vi "log analysis_gps.vi"() -> ()   [LabVIEW 2019] (continued)
0.0344,0.0343,0.0312,0.0792,0.0802,5.0949,0f000005,0*2ff36e63\n\t", "INSPVAXA,USB3,0,49.0,FINESTEERING,2107,283226.350,02000000,471d,15824;INS_ALIGNMENT_COMPLETE,INS_RTKFIXED,37.37108844765,126.72336703725,8.2202,22.3000,0.1175,-0.3192,-0.0049,-0.452699232,-0.802169824,288.131784608,0.2162,0.1626,0.2698,0.0571,0.0479,0.0400,0.0831,0.0841,5.0965,0f000001,0*8912b163\n\t", "INSPVAXA,USB3,0,48.5,FINESTEERING,2107,283227.350,02000000,471d,15824;INS_ALIGNMENT_COMPLETE,INS_RTKFIXED,37.37108931483,126.72336395391,8.2149,22.3000,0.1129,-0.2937,-0.0022,-0.567222074,-1.168347253,288.238962529,0.2212,0.1749,0.2808,0.0651,0.0592,0.0471,0.0869,0.0878,5.0924,0f000001,0*8f246b52\n\t", "INSPVAXA,USB3,0,48.5,FINESTEERING,2107,283227.850,02000000,471d,15824;INS_ALIGNMENT_COMPLETE,INS_RTKFIXED,37.37108976815,126.72336241064,8.2129,22.3000,0.1012,-0.2894,0.0009,-0.427491703,-1.215964317,288.177638677,0.2212,0.1749,0.2808,0.0651,0.0592,0.0471,0.0869,0.0878,5.0924,0f000001,0*ddfdf890\n\t", "INSPVAXA,USB3,0,43.5,FINESTEERING,2107,283228.350,02000000,471d,15824;INS_ALIGNMENT_COMPLETE,INS_RTKFIXED,37.37109022271,126.72336087108,8.2100,22.3000,0.0996,-0.2735,0.0003,-0.409798448,-1.329111694,287.820965193,0.2393,0.1944,0.2974,0.0761,0.0698,0.0531,0.0903,0.0914,5.0788,0f000001,0*ba2a3ea8\n\t", "INSPVAXA,USB3,0,43.5,FINESTEERING,2107,283228.850,02000000,471d,15824;INS_ALIGNMENT_COMPLETE,INS_RTKFIXED,37.37109066362,126.72335936248,8.2065,22.3000,0.0986,-0.2652,0.0020,-0.598740198,-1.345095429,287.386151451,0.2393,0.1944,0.2974,0.0761,0.0698,0.0531,0.0903,0.0914,5.0788,0f000001,0*2e7dd81d\n\t", "INSPVAXA,USB3,0,48.5,FINESTEERING,2107,283229.350,02000000,471d,15824;INS_ALIGNMENT_COMPLETE,INS_RTKFIXED,37.37109112291,126.72335786047,8.2034,22.3000,0.1037,-0.2722,0.0059,-0.580011682,-1.182180858,286.853066758,0.2680,0.2186,0.3192,0.0865,0.0782,0.0582,0.0931,0.0946,5.0540,0f000001,0*9b5ccdcf\n\t", "INSPVAXA,USB3,0,48.5,FINESTEERING,2107,283229.850,02000000,471d,15824;INS_ALIGNMENT_COMPLETE,INS_RTKFIXED,37.37109159656,126.72335634766,8.2007,22.3000,0.0997,-0.2660,0.0048,-0.505114639,-1.253978500,286.329147717,0.2680,0.2186,0.3192,0.0865,0.0782,0.0582,0.0931,0.0946,5.0540,0f000001,0*b8c54619\n\t", "INSPVAXA,USB3,0,48.5,FINESTEERING,2107,283230.850,02000000,471d,15824;INS_ALIGNMENT_COMPLETE,INS_RTKFIXED,37.37109255379,126.72335333433,8.1922,22.3000,0.1139,-0.2722,-0.0264,-0.549844601,-1.243677147,285.192352879,0.3030,0.2423,0.3452,0.0951,0.0845,0.0626,0.0951,0.0973,5.0218,0f000001,0*4712ada1\n\t", "INSPVAXA,USB3,0,47.5,FINESTEERING,2107,283231.850,02000000,471d,15824;INS_ALIGNMENT_COMPLETE,INS_RTKFIXED,37.37109356016,126.72335031478,8.1824,22.3000,0.1080,-0.2773,-0.0065,-0.427440692,-1.278596031,284.403841092,0.3386,0.2620,0.3738,0.1014,0.0883,0.0663,0.0962,0.0993,4.9874,0f000001,0*03e37570\n\t", "INSPVAXA,USB3,0,48.5,FINESTEERING,2107,283233.350,02000000,471d,15824;INS_ALIGNMENT_COMPLETE,INS_RTKFIXED,37.37109506136,126.72334582781,8.1673,22.3000,0.1059,-0.2882,-0.0129,-0.399188016,-1.308966160,283.569134485,0.3953,0.2852,0.4320,0.1083,0.0909,0.0717,0.0969,0.1016,4.9362,0f000001,0*c0c0ad69\n\t", "INSPVAXA,USB3,0,48.5,FINESTEERING,2107,283233.850,02000000,471d,15824;INS_ALIGNMENT_COMPLETE,INS_RTKFIXED,37.37109557748,126.72334434749,8.1612,22.3000,0.1020,-0.2689,-0.0118,-0.288207427,-1.260427493,283.382499321,0.3953,0.2852,0.4320,0.1083,0.0909,0.0717,0.0969,0.1016,4.9362,0f000001,0*9cae95f0\n\t", "INSPVAXA,USB3,0,40.5,FINESTEERING,2107,283234.350,02000000,471d,15824;INS_ALIGNMENT_COMPLETE,INS_RTKFIXED,37.37109597071,126.72334335857,8.1556,22.3000,0.0926,-0.1801,-0.0168,-0.385399344,-0.992179167,283.170226692,0.4136,0.2904,0.4588,0.1097,0.0911,0.0735,0.0969,0.1021,4.9239,0f000001,0*8e2cf425\n\t", "INSPVAXA,USB3,0,44.5,FINESTEERING,2107,283235.350,02000000,471d,15824;INS_ALIGNMENT_COMPLETE,INS_RTKFIXED,37.37109700062,126.72334017325,8.1414,22.3000,0.1228,-0.2164,-0.0234,-0.044307272,-1.163346566,282.981780278,0.4261,0.2932,0.4825,0.1104,0.0912,0.0747,0.0969,0.1023,4.9187,0f000001,0*f944742e\n\t", "INSPVAXA,USB3,0,44.5,FINESTEERING,2107,283235.850,02000000,471d,15824;INS_ALIGNMENT_COMPLETE,INS_RTKFIXED,37.37109748848,126.72333864124,8.1345,22.3000,0.1343,-0.2501,-0.0261,0.047074074,-1.173722020,282.896627938,0.4261,0.2932,0.4825,0.1104,0.0912,0.0747,0.0969,0.1023,4.9187,0f000001,0*d201ba2d\n\t", "INSPVAXA,USB3,0,49.0,FINESTEERING,2107,283236.350,02000000,471d,15824;INS_ALIGNMENT_COMPLETE,INS_RTKFIXED,37.37109796118,126.72333710973,8.1282,22.3000,0.1356,-0.2699,-0.0252,0.117707289,-1.086574547,282.783735366,0.4343,0.2946,0.5028,0.1112,0.0912,0.0756,0.0969,0.1025,4.9173,0f000001,0*2a8403f7\n\t", "INSPVAXA,USB3,0,49.0,FINESTEERING,2107,283236.850,02000000,471d,15824;INS_ALIGNMENT_COMPLETE,INS_RTKFIXED,37.37109843766,126.72333556115,8.1224,22.3000,0.1364,-0.2752,-0.0170,0.206554754,-1.115785286,282.668706587,0.4343,0.2946,0.5028,0.1112,0.0912,0.0756,0.0969,0.1025,4.9173,0f000001,0*f32b757d\n\t", "INSPVAXA,USB3,0,50.0,FINESTEERING,2107,283237.350,02000000,471d,15824;INS_ALIGNMENT_COMPLETE,INS_RTKFIXED,37.37109889709,126.72333402852,8.1172,22.3000,0.1302,-0.2622,-0.0159,0.272964655,-0.969484685,282.581344879,0.4398,0.2952,0.5196,0.1116,0.0914,0.0761,0.0969,0.1026,4.9185,0f000001,0*477c8ced\n\t", "INSPVAXA,USB3,0,50.0,FINESTEERING,2107,283237.850,02000000,471d,15824;INS_ALIGNMENT_COMPLETE,INS_RTKFIXED,37.37109934536,126.72333248224,8.1121,22.3000,0.1280,-0.2768,-0.0138,0.258054665,-1.050370160,282.484517090,0.4398,0.2952,0.5196,0.1116,0.0914,0.0761,0.0969,0.1026,4.9185,0f000001,0*cd2f787f\n\t", "INSPVAXA,USB3,0,51.5,FINESTEERING,2107,283238.350,02000000,471d,15824;INS_ALIGNMENT_COMPLETE,INS_RTKFIXED,37.37109977982,126.72333093578,8.1070,22.3000,0.1223,-0.2761,-0.0142,0.234355283,-1.035161651,282.464995705,0.4436,0.2955,0.5329,0.1118,0.0916,0.0764,0.0970,0.1026,4.9197,0f000001,0*b2aac9f1\n\t", "INSPVAXA,USB3,0,51.5,FINESTEERING,2107,283238.850,02000000,471d,15824;INS_ALIGNMENT_COMPLETE,INS_RTKFIXED,37.37110022418,126.72332937535,8.1011,22.3000,0.1168,-0.2700,-0.0206,0.387659618,-1.151934969,282.487408850,0.4436,0.2955,0.5329,0.1118,0.0916,0.0764,0.0970,0.1026,4.9197,0f000001,0*91317f18\n\t", "INSPVAXA,USB3,0,49.0,FINESTEERING,2107,283239.350,02000000,471d,15824;INS_ALIGNMENT_COMPLETE,INS_RTKFIXED,37.37110063479,126.72332783214,8.0954,22.3000,0.1184,-0.2911,-0.0146,0.524963643,-1.181982568,282.530354498,0.4459,0.2956,0.5431,0.1123,0.0918,0.0765,0.0970,0.1026,4.9196,0f000001,0*aac06e63\n\t", "INSPVAXA,USB3,0,49.0,FINESTEERING,2107,283239.850,02000000,471d,15824;INS_ALIGNMENT_COMPLETE,INS_RTKFIXED,37.37110101931,126.72332626888,8.0896,22.3000,0.1173,-0.2983,-0.0228,0.347504334,-1.218326130,282.608811447,0.4459,0.2956,0.5431,0.1123,0.0918,0.0765,0.0970,0.1026,4.9196,0f000001,0*aaab564a\n\t", "INSPVAXA,USB3,0,49.5,FINESTEERING,2107,283240.350,02000000,471d,15824;INS_ALIGNMENT_COMPLETE,INS_RTKFIXED,37.37110139226,126.72332471479,8.0839,22.3000,0.1052,-0.2558,-0.0218,0.111794667,-1.199195640,282.711507437,0.4475,0.2957,0.5507,0.1121,0.0921,0.0765,0.0971,0.1026,4.9179,0f000001,0*067ad1f3\n\t", "INSPVAXA,USB3,0,49.5,FINESTEERING,2107,283240.850,02000000,471d,15824;INS_ALIGNMENT_COMPLETE,INS_RTKFIXED,37.37110178506,126.72332315971,8.0792,22.3000,0.1224,-0.2728,-0.0239,0.192223977,-1.143692824,282.808782455,0.4475,0.2957,0.5507,0.1121,0.0921,0.0765,0.0971,0.1026,4.9179,0f000001,0*4c669a89\n\t", "INSPVAXA,USB3,0,46.0,FINESTEERING,2107,283241.350,02000000,471d,15824;INS_ALIGNMENT_COMPLETE,INS_RTKFIXED,37.37110216671,126.72332169027,8.0740,22.3000,0.1256,-0.2749,-0.0357,0.303484738,-0.991943095,282.906858014,0.4483,0.2959,0.5565,0.1130,0.0923,0.0766,0.0971,0.1026,4.9153,0f000001,0*4b7c655e\n\t", "INSPVAXA,USB3,0,49.5,FINESTEERING,2107,283242.350,02000000,471d,15824;INS_ALIGNMENT_COMPLETE,INS_RTKFIXED,37.37110294523,126.72331868826,8.0634,22.3000,0.1292,-0.2803,-0.0380,0.123672513,-0.689289621,283.242371954,0.4492,0.2961,0.5604,0.1137,0.0926,0.0766,0.0971,0.1026,4.9113,0f000001,0*f9b22440\n\t", "INSPVAXA,USB3,0,49.5,FINESTEERING,2107,283242.850,02000000,471d,15824;INS_ALIGNMENT_COMPLETE,INS_RTKFIXED,37.37110335770,126.72331719520,8.0593,22.3000,0.1255,-0.2698,-0.0380,0.121355626,-0.605377000,283.439898811,0.4492,0.2961,0.5604,0.1137,0.0926,0.0766,0.0971,0.1026,4.9113,0f000001,0*de8b7806\n\t", "INSPVAXA,USB3,0,49.0,FINESTEERING,2107,283244.350,02008000,471d,15824;INS_ALIGNMENT_COMPLETE,INS_RTKFIXED,37.37110468880,126.72331252353,8.0457,22.3000,0.1303,-0.2564,-0.0224,0.139221287,-0.844011919,284.159794533,0.4505,0.2963,0.5646,0.1137,0.0927,0.0766,0.0971,0.1025,4.8983,0f000001,0*7deeba4a\n\t", "INSPVAXA,USB3,0,49.0,FINESTEERING,2107,283244.850,02008000,471d,15824;INS_ALIGNMENT_COMPLETE,INS_RTKFIXED,37.37110513730,126.72331104111,8.0417,22.3000,0.1309,-0.2685,-0.0243,0.209910171,-0.848689827,284.605167035,0.4505,0.2963,0.5646,0.1137,0.0927,0.0766,0.0971,0.1025,4.8983,0f000001,0*e4fb8053\n\t", "INSPVAXA,USB3,0,50.0,FINESTEERING,2107,283245.350,02008000,471d,15824;INS_ALIGNMENT_COMPLETE,INS_RTKFIXED,37.37110557782,126.72330954830,8.0387,22.3000,0.1426,-0.2572,-0.0360,0.139361200,-0.921723778,285.121059969,0.4506,0.2964,0.5656,0.1138,0.0927,0.0767,0.0971,0.1024,4.8921,0f000001,0*fcb5f941\n\t", "INSPVAXA,USB3,0,48.5,FINESTEERING,2107,283246.350,02008000,471d,15824;INS_ALIGNMENT_COMPLETE,INS_RTKFIXED,37.37110650296,126.72330657394,8.0329,22.3000,0.1463,-0.2502,-0.0217,0.213692795,-0.911589097,286.397564613,0.4505,0.2965,0.5663,0.1141,0.0927,0.0768,0.0971,0.1023,4.8873,0f000001,0*feddfe3b\n\t", "INSPVAXA,USB3,0,48.5,FINESTEERING,2107,283246.850,02008000,471d,15824;INS_ALIGNMENT_COMPLETE,INS_RTKFIXED,37.37110698644,126.72330510005,8.0315,22.3000,0.1343,-0.2488,-0.0293,0.310721762,-0.889438345,287.090761589,0.4505,0.2965,0.5663,0.1141,0.0927,0.0768,0.0971,0.1023,4.8873,0f000001,0*ee8d45a4\n\t", "INSPVAXA,USB3,0,47.0,FINESTEERING,2107,283247.350,02008000,471d,15824;INS_ALIGNMENT_COMPLETE,INS_RTKFIXED,37.37110746549,126.72330361825,8.0305,22.3000,0.1318,-0.2455,-0.0310,0.265513660,-1.003037989,287.732787222,0.4503,0.2965,0.5665,0.1141,0.0927,0.0768,0.0970,0.1023,4.8832,0f000001,0*16257acc\n\t", "INSPVAXA,USB3,0,51.5,FINESTEERING,2107,283248.350,02008000,471d,15824;INS_ALIGNMENT_COMPLETE,INS_RTKFIXED,37.37110841164,126.72330070273,8.0292,22.3000,0.1212,-0.2566,-0.0210,0.033040840,-0.857112226,288.813321277,0.4501,0.2965,0.5666,0.1141,0.0927,0.0770,0.0970,0.1022,4.8803,0f000001,0*d8465b23\n\t", "INSPVAXA,USB3,0,48.5,FINESTEERING,2107,283249.850,02008000,471d,15824;INS_ALIGNMENT_COMPLETE,INS_RTKFIXED,37.37110988356,126.72329635950,8.0261,22.3000,0.1256,-0.2402,-0.0147,0.060845598,-0.557595115,289.806680124,0.4499,0.2965,0.5665,0.1144,0.0927,0.0771,0.0970,0.1022,4.8781,0f000001,0*763984e0\n\t", "INSPVAXA,USB3,0,49.5,FINESTEERING,2107,283250.350,02000000,471d,15824;INS_ALIGNMENT_COMPLETE,INS_RTKFIXED,37.37111038564,126.72329491003,8.0267,22.3000,0.1228,-0.2382,-0.0157,-0.018569181,-0.488431655,290.019315132,0.4500,0.2966,0.5665,0.1143,0.0928,0.0772,0.0970,0.1022,4.8762,0f000001,0*c58162f6\n\t", "INSPVAXA,USB3,0,49.5,FINESTEERING,2107,283251.850,02000000,471d,15824;INS_ALIGNMENT_COMPLETE,INS_RTKFIXED,37.37111192959,126.72329056644,8.0317,22.3000,0.1243,-0.2388,-0.0145,-0.052610032,-0.761049634,290.503776347,0.4499,0.2966,0.5666,0.1142,0.0928,0.0773,0.0970,0.1021,4.8746,0f000001,0*ba4c3e6a\n\t", "INSPVAXA,USB3,0,49.5,FINESTEERING,2107,283252.350,02000000,471d,15824;INS_ALIGNMENT_COMPLETE,INS_RTKFIXED,37.37111241968,126.72328920118,8.0341,22.3000,0.1282,-0.2523,-0.0162,-0.150683297,-0.978077835,290.683925037,0.4496,0.2967,0.5667,0.1142,0.0928,0.0774,0.0970,0.1021,4.8737,0f000001,0*23232e95\n\t", "INSPVAXA,USB3,0,50.0,FINESTEERING,2107,283253.850,02000000,471d,15824;INS_ALIGNMENT_COMPLETE,INS_RTKFIXED,37.37111392592,126.72328504795,8.0397,22.3000,0.1448,-0.2935,-0.0163,-0.197937020,-0.955376116,291.000430762,0.4494,0.2968,0.5669,0.1142,0.0929,0.0775,0.0970,0.1021,4.8734,0f000001,0*886ef4ee\n\t", "INSPVAXA,USB3,0,47.0,FINESTEERING,2107,283256.350,02000000,471d,15824;INS_ALIGNMENT_COMPLETE,INS_RTKFIXED,37.37111667800,126.72327759739,8.0487,22.3000,0.1131,-0.2631,-0.0127,-0.014268903,-1.510864451,290.200992248,0.4483,0.2970,0.5675,0.1142,0.0929,0.0778,0.0970,0.1021,4.8754,0f000001,0*3c5e786f\n\t", "INSPVAXA,USB3,0,44.0,FINESTEERING,2107,283276.900,02000000,471d,15824;INS_ALIGNMENT_COMPLETE,INS_RTKFIXED,37.37113577898,126.72321589270,7.9963,22.3000,0.1042,-0.2583,-0.0142,-0.525742005,-1.010949392,284.316907769,0.4477,0.2970,0.5693,0.1141,0.0929,0.0780,0.0969,0.1021,4.9003,0f000001,0*b42fff2f\n\t", "INSPVAXA,USB3,0,47.5,FINESTEERING,2107,283277.900,02000000,471d,15824;INS_ALIGNMENT_COMPLETE,INS_RTKFIXED,37.37113658418,126.72321294940,7.9963,22.3000,0.0900,-0.2507,-0.0130,-0.397975122,-0.687807065,284.132829935,0.4476,0.2970,0.5692,0.1141,0.0929,0.0780,0.0969,0.1021,4.9017,0f000001,0*e88e7117\n\t", "INSPVAXA,USB3,0,48.0,FINESTEERING,2107,283279.400,02000000,471d,15824;INS_ALIGNMENT_COMPLETE,INS_RTKFIXED,37.37113775239,126.72320841739,7.9941,22.3000,0.0997,-0.2552,-0.0140,-0.507226746,-0.753730833,284.120099148,0.4481,0.2971,0.5694,0.1142,0.0928,0.0780,0.0969,0.1021,4.9040,0f000001,0*1d440196\n\t", "INSPVAXA,USB3,0,49.5,FINESTEERING,2107,283281.400,02000000,471d,15824;INS_ALIGNMENT_COMPLETE,INS_RTKFIXED,37.37113937207,126.72320229897,7.9921,22.3000,0.0832,-0.2611,-0.0143,-0.573096548,-0.909868573,284.165048220,0.4480,0.2971,0.5695,0.1141,0.0928,0.0780,0.0969,0.1020,4.9063,0f000001,0*a447e184\n\t", "INSPVAXA,USB3,0,46.5,FINESTEERING,2107,283282.400,02000000,471d,15824;INS_ALIGNMENT_COMPLETE,INS_RTKFIXED,37.37114019228,126.72319922313,7.9923,22.3000,0.0951,-0.2773,-0.0041,-0.536108170,-0.972919730,284.196085514,0.4479,0.2971,0.5695,0.1142,0.0928,0.0780,0.0969,0.1020,4.9076,0f000001,0*84139aa4\n\t", "INSPVAXA,USB3,0,46.5,FINESTEERING,2107,283282.900,02000000,471d,15824;INS_ALIGNMENT_COMPLETE,INS_RTKFIXED,37.37114058950,126.72319773387,7.9934,22.3000,0.0877,-0.2549,-0.0017,-0.494597000,-1.027505059,284.193699640,0.4479,0.2971,0.5695,0.1142,0.0928,0.0780,0.0969,0.1020,4.9076,0f000001,0*ecacd8f3\n\t", "INSPVAXA,USB3,0,45.5,FINESTEERING,2107,283284.400,02000000,471d,15824;INS_ALIGNMENT_COMPLETE,INS_RTKFIXED,37.37114183564,126.72319312332,7.9966,22.3000,0.0813,-0.2603,0.0021,-0.541869353,-0.903555569,284.232610240,0.4477,0.2970,0.5694,0.1142,0.0928,0.0780,0.0969,0.1020,4.9102,0f000001,0*cca71bea\n\t", "INSPVAXA,USB3,0,48.5,FINESTEERING,2107,283285.400,02000000,471d,15824;INS_ALIGNMENT_COMPLETE,INS_RTKFIXED,37.37114271022,126.72319003823,7.9928,22.3000,0.0833,-0.2558,0.0046,-0.428723996,-1.048111002,284.209543070,0.4481,0.2971,0.5696,0.1142,0.0929,0.0780,0.0969,0.1020,4.9114,0f000001,0*c956834d\n\t", "INSPVAXA,USB3,0,48.5,FINESTEERING,2107,283287.900,02000000,471d,15824;INS_ALIGNMENT_COMPLETE,INS_RTKFIXED,37.37114488961,126.72318257858,7.9892,22.3000,0.0816,-0.2710,-0.0129,-0.307821910,-0.791572472,283.812578734,0.4475,0.2971,0.5695,0.1142,0.0928,0.0780,0.0969,0.1020,4.9139,0f000001,0*ad245747\n\t", "INSPVAXA,USB3,0,49.0,FINESTEERING,2107,283290.400,02000000,471d,15824;INS_ALIGNMENT_COMPLETE,INS_RTKFIXED,37.37114696201,126.72317494055,7.9797,22.3000,0.0686,-0.2611,-0.0031,-0.360570478,-0.610945799,282.620180984,0.4490,0.2972,0.5701,0.1142,0.0929,0.0781,0.0969,0.1020,4.9167,0f000001,0*1d53d3bd\n\t", "INSPVAXA,USB3,0,45.5,FINESTEERING,2107,283291.400,02000000,471d,15824;INS_ALIGNMENT_COMPLETE,INS_RTKFIXED,37.37114777556,126.72317182162,7.9735,22.3000,0.0763,-0.2712,-0.0094,-0.152974893,-0.616653887,282.239897550,0.4489,0.2971,0.5701,0.1142,0.0928,0.0781,0.0969,0.1020,4.9171,0f000001,0*c60dfbfa\n\t", "INSPVAXA,USB3,0,45.0,FINESTEERING,2107,283292.900,02008000,471d,15824;INS_ALIGNMENT_COMPLETE,INS_RTKFIXED,37.37114893041,126.72316711689,7.9673,22.3000,0.0793,-0.2669,-0.0229,-0.307538430,-0.866474135,281.723711903,0.4489,0.2972,0.5701,0.1141,0.0929,0.0781,0.0969,0.1020,4.9176,0f000001,0*1a68f6c8\n\t", "INSPVAXA,USB3,0,46.5,FINESTEERING,2107,283293.400,02008000,471d,15824;INS_ALIGNMENT_COMPLETE,INS_RTKFIXED,37.37114931460,126.72316558102,7.9656,22.3000,0.0841,-0.2703,-0.0190,-0.304587768,-0.848212966,281.590040243,0.4485,0.2971,0.5701,0.1141,0.0929,0.0781,0.0969,0.1020,4.9184,0f000001,0*b7765035\n\t", "INSPVAXA,USB3,0,46.5,FINESTEERING,2107,283293.900,02008000,471d,15824;INS_ALIGNMENT_COMPLETE,INS_RTKFIXED,37.37114971165,126.72316402474,7.9632,22.3000,0.0893,-0.2652,-0.0218,-0.263902472,-0.725819533,281.502254462,0.4485,0.2971,0.5701,0.1141,0.0929,0.0781,0.0969,0.1020,4.9184,0f000001,0*152a6832\n\t", "DUALANTENNAHEADINGA,USB3,0,47.5,FINESTEERING,2107,283294.400,02008000,d426,15824;SOL_COMPUTED,L1_FLOAT,-1.000000000,239.844818115,64.606910706,0.0,166.616958618,114.780426025,\"631T\",14,7,7,7,04,00,20,23*19bdebe6\n\t", "INSPVAXA,USB3,0,47.5,FINESTEERING,2107,283294.900,02008000,471d,15824;INS_ALIGNMENT_COMPLETE,INS_RTKFIXED,37.37115047180,126.72316089302,7.9563,22.3000,0.0884,-0.2648,-0.0252,-0.144222363,-0.665231738,281.410020800,0.4483,0.2971,0.5702,0.1141,0.0929,0.0781,0.0969,0.1020,4.9194,0f000001,0*3b62bb88\n\t", "INSPVAXA,USB3,0,50.0,FINESTEERING,2107,283295.400,02008000,471d,15824;INS_ALIGNMENT_COMPLETE,INS_RTKFIXED,37.37115084282,126.72315933978,7.9528,22.3000,0.0924,-0.2759,-0.0196,-0.193072423,-0.599159987,281.404191398,0.4483,0.2972,0.5704,0.1141,0.0929,0.0781,0.0969,0.1020,4.9206,0f000001,0*10d0b358\n\t", "DUALANTENNAHEADINGA,USB3,0,50.0,FINESTEERING,2107,283295.900,02008000,d426,15824;SOL_COMPUTED,L1_FLOAT,-1.000000000,237.505355835,63.904857635,0.0,132.502212524,100.132637024,\"631T\",18,7,7,7,04,00,20,23*65892cbe\n\t", "INSPVAXA,USB3,0,48.0,FINESTEERING,2107,283296.400,02000000,471d,15824;INS_ALIGNMENT_COMPLETE,INS_RTKFIXED,37.37115159718,126.72315615738,7.9465,22.3000,0.0791,-0.2694,-0.0207,-0.243399064,-0.670303130,281.350381615,0.4482,0.2972,0.5704,0.1141,0.0929,0.0781,0.0969,0.1020,4.9219,0f000001,0*42d4064f\n\t", "DUALANTENNAHEADINGA,USB3,0,48.0,FINESTEERING,2107,283296.900,02000000,d426,15824;SOL_COMPUTED,L1_FLOAT,-1.000000000,239.343627930,64.402900696,0.0,148.477706909,103.162033081,\"631T\",15,7,7,7,04,00,20,23*e8ad3b91\n\t", "INSPVAXA,USB3,0,48.5,FINESTEERING,2107,283297.400,02000000,471d,15824;INS_ALIGNMENT_COMPLETE,INS_RTKFIXED,37.37115233691,126.72315301561,7.9394,22.3000,0.0884,-0.2678,-0.0159,-0.231727201,-0.925475232,281.406187486,0.4479,0.2972,0.5705,0.1141,0.0929,0.0781,0.0969,0.1020,4.9234,0f000001,0*12bb3ab8\n\t", "INSPVAXA,USB3,0,48.5,FINESTEERING,2107,283297.900,02000000,471d,15824;INS_ALIGNMENT_COMPLETE,INS_RTKFIXED,37.37115269099,126.72315144073,7.9365,22.3000,0.0910,-0.2656,-0.0151,-0.313313206,-1.052318867,281.426390145,0.4479,0.2972,0.5705,0.1141,0.0929,0.0781,0.0969,0.1020,4.9234,0f000001,0*736ed8bf\n\t", "INSPVAXA,USB3,0,51.0,FINESTEERING,2107,283298.400,02008000,471d,15824;INS_ALIGNMENT_COMPLETE,INS_RTKFIXED,37.37115305235,126.72314988342,7.9353,22.3000,0.0916,-0.2769,-0.0209,-0.334551062,-1.062649728,281.510450762,0.4462,0.2970,0.5704,0.1139,0.0928,0.0781,0.0969,0.1019,4.9249,0f000001,0*7ea0d7b1\n\t", "INSPVAXA,USB3,0,51.0,FINESTEERING,2107,283298.900,02008000,471d,15824;INS_ALIGNMENT_COMPLETE,INS_RTKFIXED,37.37115341393,126.72314832428,7.9330,22.3000,0.0837,-0.2625,-0.0169,-0.397478234,-1.037439092,281.585618235,0.4462,0.2970,0.5704,0.1139,0.0928,0.0781,0.0969,0.1019,4.9249,0f000001,0*addaa3c1\n\t", "INSPVAXA,USB3,0,45.0,FINESTEERING,2107,283299.400,02008000,471d,15824;INS_ALIGNMENT_COMPLETE,INS_RTKFIXED,37.37115377370,126.72314676184,7.9298,22.3000,0.0909,-0.2631,-0.0145,-0.362966216,-0.969827593,281.677827339,0.4450,0.2970,0.5703,0.1138,0.0928,0.0781,0.0969,0.1019,4.9264,0f000001,0*1c473296\n\t", "INSPVAXA,USB3,0,45.0,FINESTEERING,2107,283299.900,02008000,471d,15824;INS_ALIGNMENT_COMPLETE,INS_RTKFIXED,37.37115412853,126.72314521703,7.9265,22.3000,0.0831,-0.2721,-0.0168,-0.334055092,-0.857613920,281.755753897,0.4450,0.2970,0.5703,0.1138,0.0928,0.0781,0.0969,0.1019,4.9264,0f000001,0*4d7a0a60\n\t", "DUALANTENNAHEADINGA,USB3,0,40.5,FINESTEERING,2107,283300.400,02008000,d426,15824;SOL_COMPUTED,L1_FLOAT,-1.000000000,232.358734131,64.946899414,0.0,184.697021484,151.855468750,\"631T\",13,5,5,5,04,00,20,03*f60c6ef8\n\t", "INSPVAXA,USB3,0,40.5,FINESTEERING,2107,283300.900,02008000,471d,15824;INS_ALIGNMENT_COMPLETE,INS_RTKFIXED,37.37115484988,126.72314211300,7.9189,22.3000,0.0947,-0.2610,-0.0185,-0.569818245,-0.847887628,281.897603844,0.4441,0.2969,0.5702,0.1137,0.0928,0.0781,0.0969,0.1019,4.9278,0f000001,0*956f8967\n\t", "DUALANTENNAHEADINGA,USB3,0,48.5,FINESTEERING,2107,283301.400,02008000,d426,15824;SOL_COMPUTED,L1_FLOAT,-1.000000000,241.477539063,62.723838806,0.0,360.000000000,180.000000000,\"631T\",17,6,6,5,04,00,20,03*c892e55f\n\t", "INSPVAXA,USB3,0,48.5,FINESTEERING,2107,283301.900,02008000,471d,15824;INS_ALIGNMENT_COMPLETE,INS_RTKFIXED,37.37115557070,126.72313902980,7.9130,22.3000,0.0918,-0.2789,-0.0166,-0.521820330,-0.769982441,282.107376455,0.4435,0.2967,0.5700,0.1137,0.0928,0.0780,0.0969,0.1019,4.9292,0f000001,0*6ce7102f\n\t", "DUALANTENNAHEADINGA,USB3,0,45.0,FINESTEERING,2107,283302.400,02000000,d426,15824;SOL_COMPUTED,NARROW_FLOAT,-1.000000000,244.334762573,52.398559570,0.0,117.969345093,144.888336182,\"631T\",16,7,7,5,04,00,20,03*fc904e6e\n\t", "INSPVAXA,USB3,0,45.0,FINESTEERING,2107,283302.900,02000000,471d,15824;INS_ALIGNMENT_COMPLETE,INS_RTKFIXED,37.37115630629,126.72313591072,7.9093,22.3000,0.0953,-0.2572,-0.0206,-0.734868451,-0.639941335,282.297303712,0.4435,0.2967,0.5699,0.1137,0.0928,0.0780,0.0969,0.1019,4.9307,0f000001,0*e76bd6df\n\t", "DUALANTENNAHEADINGA,USB3,0,47.0,FINESTEERING,2107,283303.400,02000000,d426,15824;SOL_COMPUTED,NARROW_FLOAT,-1.000000000,231.882415771,63.058189392,0.0,139.197525024,151.772613525,\"631T\",16,5,5,5,04,00,20,03*97a548ee\n\t", "DUALANTENNAHEADINGA,USB3,0,47.0,FINESTEERING,2107,283303.900,02000000,d426,15824;SOL_COMPUTED,NARROW_FLOAT,-1.000000000,232.017898560,63.345188141,0.0,143.997665405,156.088058472,\"631T\",16,5,5,5,04,00,20,03*4eb7c41d\n\t", "DUALANTENNAHEADINGA,USB3,0,48.5,FINESTEERING,2107,283304.400,02000000,d426,15824;SOL_COMPUTED,NARROW_FLOAT,-1.000000000,234.068984985,56.849258423,0.0,140.735427856,121.552192688,\"631T\",17,5,5,5,04,00,20,03*01bf1f6c\n\t", "DUALANTENNAHEADINGA,USB3,0,48.5,FINESTEERING,2107,283304.900,02000000,d426,15824;SOL_COMPUTED,NARROW_FLOAT,-1.000000000,233.255889893,60.512351990,0.0,144.115737915,132.290557861,\"631T\",16,5,5,5,04,00,20,03*f75e5353\n\t", "DUALANTENNAHEADINGA,USB3,0,44.5,FINESTEERING,2107,283305.400,02000000,d426,15824;SOL_COMPUTED,L1_FLOAT,-1.000000000,233.577301025,62.029331207,0.0,96.220359802,93.397712708,\"631T\",16,7,7,7,04,00,20,23*c706f208\n\t", "INSPVAXA,USB3,0,44.5,FINESTEERING,2107,283305.900,02000000,471d,15824;INS_ALIGNMENT_COMPLETE,INS_RTKFIXED,37.37115859876,126.72312661710,7.8931,22.3000,0.1099,-0.2740,-0.0203,-0.656948256,-1.026367875,282.954540739,0.4425,0.2966,0.5699,0.1135,0.0928,0.0781,0.0969,0.1019,4.9352,0f000001,0*1036819f\n\t", "INSPVAXA,USB3,0,46.0,FINESTEERING,2107,283306.400,02000000,471d,15824;INS_ALIGNMENT_COMPLETE,INS_RTKFIXED,37.37115900607,126.72312505339,7.8906,22.3000,0.1023,-0.2590,-0.0088,-0.729755856,-0.991327680,283.031299581,0.4419,0.2965,0.5696,0.1135,0.0928,0.0780,0.0969,0.1019,4.9367,0f000001,0*5e887597\n\t", "DUALANTENNAHEADINGA,USB3,0,46.0,FINESTEERING,2107,283306.900,02000000,d426,15824;SOL_COMPUTED,L1_FLOAT,-1.000000000,239.290145874,67.008094788,0.0,195.596420288,134.664169312,\"631T\",14,5,5,5,04,00,20,03*267cdbf0\n\t", "DUALANTENNAHEADINGA,USB3,0,49.5,FINESTEERING,2107,283307.400,02000000,d426,15824;SOL_COMPUTED,L1_FLOAT,-1.000000000,232.261947632,66.446723938,0.0,159.915008545,144.811691284,\"631T\",14,5,5,5,04,00,20,03*cd69fe68\n\t", "DUALANTENNAHEADINGA,USB3,0,49.5,FINESTEERING,2107,283307.900,02000000,d426,15824;SOL_COMPUTED,L1_FLOAT,-1.000000000,232.562942505,64.960189819,0.0,154.937866211,134.466018677,\"631T\",15,5,5,5,04,00,20,03*e7f8f672\n\t", "DUALANTENNAHEADINGA,USB3,0,51.0,FINESTEERING,2107,283308.400,02000000,d426,15824;SOL_COMPUTED,L1_FLOAT,-1.000000000,235.060028076,63.952377319,0.0,259.231262207,169.746810913,\"631T\",15,5,5,5,04,00,20,03*f7293e70\n\t", "INSPVAXA,USB3,0,51.0,FINESTEERING,2107,283308.900,02000000,471d,15824;INS_ALIGNMENT_COMPLETE,INS_RTKFIXED,37.37116096041,126.72311737455,7.8778,22.3000,0.0846,-0.2672,-0.0151,-0.781249790,-0.507158310,282.995006932,0.4410,0.2964,0.5694,0.1133,0.0927,0.0780,0.0968,0.1018,4.9395,0f000001,0*4118e416\n\t", "INSPVAXA,USB3,0,47.5,FINESTEERING,2107,283309.400,02000000,471d,15824;INS_ALIGNMENT_COMPLETE,INS_RTKFIXED,37.37116135505,126.72311582888,7.8756,22.3000,0.0948,-0.2836,-0.0131,-0.715867261,-0.524623551,282.915298910,0.4409,0.2962,0.5692,0.1133,0.0927,0.0780,0.0968,0.1018,4.9410,0f000001,0*81cbe5cb\n\t", "INSPVAXA,USB3,0,47.5,FINESTEERING,2107,283309.900,02000000,471d,15824;INS_ALIGNMENT_COMPLETE,INS_RTKFIXED,37.37116173975,126.72311427706,7.8728,22.3000,0.0962,-0.2788,-0.0165,-0.819724442,-0.652921379,282.793511775,0.4409,0.2962,0.5692,0.1133,0.0927,0.0780,0.0968,0.1018,4.9410,0f000001,0*d0f32b82\n\t", "DUALANTENNAHEADINGA,USB3,0,49.5,FINESTEERING,2107,283310.400,02000000,d426,15824;SOL_COMPUTED,NARROW_FLOAT,-1.000000000,251.362304688,59.888744354,0.0,206.856552124,155.140167236,\"631T\",17,7,7,5,04,00,20,03*1094d047\n\t", "DUALANTENNAHEADINGA,USB3,0,49.5,FINESTEERING,2107,283310.900,02000000,d426,15824;SOL_COMPUTED,NARROW_FLOAT,-1.000000000,251.351150513,59.773147583,0.0,206.432357788,155.578613281,\"631T\",16,7,7,5,04,00,20,03*7af03570\n\t", "INSPVAXA,USB3,0,48.0,FINESTEERING,2107,283311.400,02000000,471d,15824;INS_ALIGNMENT_COMPLETE,INS_RTKFIXED,37.37116288417,126.72310962036,7.8652,22.3000,0.0869,-0.2743,-0.0174,-0.761855040,-0.888417271,282.272425942,0.4407,0.2962,0.5691,0.1131,0.0927,0.0780,0.0968,0.1018,4.9438,0f000001,0*0cfd0bf9\n\t", "DUALANTENNAHEADINGA,USB3,0,48.0,FINESTEERING,2107,283311.900,02000000,d426,15824;SOL_COMPUTED,NARROW_FLOAT,-1.000000000,256.476898193,63.091281891,0.0,360.000000000,180.000000000,\"631T\",16,6,6,5,04,00,20,03*76034569\n\t", "DUALANTENNAHEADINGA,USB3,0,47.0,FINESTEERING,2107,283312.400,02000000,d426,15824;SOL_COMPUTED,L1_FLOAT,-1.000000000,236.672042847,63.326492310,0.0,146.049911499,114.689262390,\"631T\",17,5,5,5,04,00,20,03*2d6dda53\n\t", "DUALANTENNAHEADINGA,USB3,0,47.0,FINESTEERING,2107,283312.900,02000000,d426,15824;SOL_COMPUTED,L1_FLOAT,-1.000000000,236.406433105,63.618362427,0.0,144.065521240,114.259201050,\"631T\",19,5,5,5,04,00,20,03*a0545f5a\n\t", "DUALANTENNAHEADINGA,USB3,0,48.0,FINESTEERING,2107,283313.400,02000000,d426,15824;SOL_COMPUTED,NARROW_FLOAT,-1.000000000,249.966949463,62.680927277,0.0,300.232086182,155.331420898,\"631T\",19,8,8,6,04,00,20,23*b56427c2\n\t", "DUALANTENNAHEADINGA,USB3,0,48.0,FINESTEERING,2107,283313.900,02000000,d426,15824;SOL_COMPUTED,NARROW_FLOAT,-1.000000000,249.735733032,62.666515350,0.0,296.963775635,155.122772217,\"631T\",17,8,8,7,04,00,20,23*38c36f09\n\t", "DUALANTENNAHEADINGA,USB3,0,48.0,FINESTEERING,2107,283314.400,02000000,d426,15824;SOL_COMPUTED,L1_FLOAT,-1.000000000,262.029388428,61.695976257,0.0,360.000000000,162.501907349,\"631T\",16,8,8,7,04,00,20,23*1cdc20bd\n\t", "DUALANTENNAHEADINGA,USB3,0,48.0,FINESTEERING,2107,283314.900,02000000,d426,15824;SOL_COMPUTED,L1_FLOAT,-1.000000000,261.856536865,61.556816101,0.0,360.000000000,163.368423462,\"631T\",15,8,8,7,04,00,20,23*198a35c5\n\t", "DUALANTENNAHEADINGA,USB3,0,49.0,FINESTEERING,2107,283315.400,02000000,d426,15824;SOL_COMPUTED,L1_FLOAT,-1.000000000,241.071945190,70.013267517,0.0,216.117965698,130.788757324,\"631T\",14,7,7,7,04,00,20,23*ac92fc81\n\t", "DUALANTENNAHEADINGA,USB3,0,49.0,FINESTEERING,2107,283315.900,02000000,d426,15824;SOL_COMPUTED,L1_FLOAT,-1.000000000,240.838073730,70.253372192,0.0,215.071411133,130.065658569,\"631T\",14,7,7,7,04,00,20,23*360ed7d2\n\t", "DUALANTENNAHEADINGA,USB3,0,50.0,FINESTEERING,2107,283316.400,02000000,d426,15824;SOL_COMPUTED,L1_FLOAT,-1.000000000,243.607940674,69.715850830,0.0,272.601806641,140.221450806,\"631T\",14,7,7,7,04,00,20,23*51c69ef2\n\t", "DUALANTENNAHEADINGA,USB3,0,50.0,FINESTEERING,2107,283316.900,02000000,d426,15824;SOL_COMPUTED,L1_FLOAT,-1.000000000,245.043029785,68.131629944,0.0,281.695404053,144.677200317,\"631T\",15,7,7,7,04,00,20,23*f1a17a24\n\t", "DUALANTENNAHEADINGA,USB3,0,50.0,FINESTEERING,2107,283317.400,02000000,d426,15824;SOL_COMPUTED,L1_FLOAT,-1.000000000,270.938415527,64.219497681,0.0,360.000000000,166.916473389,\"631T\",15,8,8,7,04,00,20,23*09ee87ba\n\t", "DUALANTENNAHEADINGA,USB3,0,50.0,FINESTEERING,2107,283317.900,02000000,d426,15824;SOL_COMPUTED,L1_FLOAT,-1.000000000,270.609985352,63.750827789,0.0,360.000000000,169.041946411,\"631T\",17,8,8,7,04,00,20,23*f5bf3eac\n\t", "DUALANTENNAHEADINGA,USB3,0,47.5,FINESTEERING,2107,283318.400,02000000,d426,15824;SOL_COMPUTED,NARROW_FLOAT,-1.000000000,281.381378174,66.745414734,0.0,360.000000000,168.558471680,\"631T\",17,8,8,7,04,00,20,23*c33407f9\n\t", "DUALANTENNAHEADINGA,USB3,0,47.5,FINESTEERING,2107,283318.900,02000000,d426,15824;SOL_COMPUTED,NARROW_FLOAT,-1.000000000,279.926574707,66.934852600,0.0,360.000000000,167.527023315,\"631T\",17,8,8,7,04,00,20,23*f3d388f9\n\t", "DUALANTENNAHEADINGA,USB3,0,45.0,FINESTEERING,2107,283319.400,02000000,d426,15824;SOL_COMPUTED,L1_FLOAT,-1.000000000,249.257110596,70.348373413,0.0,326.773925781,134.559478760,\"631T\",16,7,7,7,04,00,20,23*e6bdd1ed\n\t", "DUALANTENNAHEADINGA,USB3,0,45.0,FINESTEERING,2107,283319.900,02000000,d426,15824;SOL_COMPUTED,L1_FLOAT,-1.000000000,248.767288208,70.954589844,0.0,326.445281982,135.310943604,\"631T\",14,5,5,5,04,00,20,03*3a82e8e8\n\t", "DUALANTENNAHEADINGA,USB3,0,46.5,FINESTEERING,2107,283320.400,02000000,d426,15824;SOL_COMPUTED,L1_FLOAT,-1.000000000,258.042144775,75.598983765,0.0,360.000000000,180.000000000,\"631T\",15,5,5,5,04,00,20,03*b6617cb0\n\t", "DUALANTENNAHEADINGA,USB3,0,46.5,FINESTEERING,2107,283320.900,02000000,d426,15824;SOL_COMPUTED,L1_FLOAT,-1.000000000,253.391662598,75.137130737,0.0,360.000000000,180.000000000,\"631T\",14,5,5,5,04,00,20,03*50d197fe\n\t", "DUALANTENNAHEADINGA,USB3,0,46.5,FINESTEERING,2107,283321.400,02000000,d426,15824;SOL_COMPUTED,L1_FLOAT,-1.000000000,312.583312988,56.468681335,0.0,360.000000000,180.000000000,\"631T\",14,6,6,5,04,00,20,03*0f80647d\n\t", "DUALANTENNAHEADINGA,USB3,0,46.5,FINESTEERING,2107,283321.900,02000000,d426,15824;SOL_COMPUTED,L1_FLOAT,-1.000000000,310.554901123,55.892704010,0.0,360.000000000,180.000000000,\"631T\",16,6,6,5,04,00,20,03*74537864\n\t", "DUALANTENNAHEADINGA,USB3,0,41.0,FINESTEERING,2107,283322.400,02008000,d426,15824;SOL_COMPUTED,L1_FLOAT,-1.000000000,241.266906738,69.189468384,0.0,360.000000000,180.000000000,\"631T\",17,5,5,5,04,00,20,03*c679f6f8\n\t", "DUALANTENNAHEADINGA,USB3,0,41.0,FINESTEERING,2107,283322.900,02008000,d426,15824;SOL_COMPUTED,L1_FLOAT,-1.000000000,239.202957153,73.481590271,0.0,360.000000000,180.000000000,\"631T\",16,5,5,5,04,00,20,03*1cc6a146\n\t", "DUALANTENNAHEADINGA,USB3,0,47.5,FINESTEERING,2107,283323.400,02008000,d426,15824;SOL_COMPUTED,L1_FLOAT,-1.000000000,238.744445801,53.518810272,0.0,151.505752563,125.381988525,\"631T\",19,6,6,5,04,00,20,03*673b97e4\n\t", "DUALANTENNAHEADINGA,USB3,0,47.5,FINESTEERING,2107,283323.900,02008000,d426,15824;SOL_COMPUTED,L1_FLOAT,-1.000000000,240.007232666,54.498615265,0.0,179.365921021,137.099334717,\"631T\",17,6,6,5,04,00,20,03*8af523f5\n\t", "DUALANTENNAHEADINGA,USB3,0,45.5,FINESTEERING,2107,283324.400,02008000,d426,15824;SOL_COMPUTED,L1_FLOAT,-1.000000000,236.690521240,63.104007721,0.0,147.733261108,120.137512207,\"631T\",18,5,5,5,04,00,20,03*a038ef34\n\t", "DUALANTENNAHEADINGA,USB3,0,45.5,FINESTEERING,2107,283324.900,02008000,d426,15824;SOL_COMPUTED,L1_FLOAT,-1.000000000,235.601470947,66.503868103,0.0,154.081848145,121.723312378,\"631T\",17,5,5,5,04,00,20,03*b1d66122\n\t", "DUALANTENNAHEADINGA,USB3,0,48.0,FINESTEERING,2107,283325.400,02008000,d426,15824;SOL_COMPUTED,NARROW_FLOAT,-1.000000000,247.574691772,57.258007050,0.0,263.334472656,160.580810547,\"631T\",14,8,8,7,04,00,20,23*fe321c1a\n\t", "DUALANTENNAHEADINGA,USB3,0,48.0,FINESTEERING,2107,283325.900,02008000,d426,15824;SOL_COMPUTED,NARROW_FLOAT,-1.000000000,247.226425171,56.712402344,0.0,254.219528198,159.121383667,\"631T\",14,8,8,7,04,00,20,23*0ca5ab8a\n\t", "DUALANTENNAHEADINGA,USB3,0,49.5,FINESTEERING,2107,283326.900,02008000,d426,15824;SOL_COMPUTED,L1_FLOAT,-1.000000000,236.025100708,66.578720093,0.0,191.472290039,141.501235962,\"631T\",15,7,7,7,04,00,20,23*59a2ecb1\n\t", "DUALANTENNAHEADINGA,USB3,0,49.5,FINESTEERING,2107,283327.900,02008000,d426,15824;SOL_COMPUTED,L1_FLOAT,-1.000000000,236.365600586,64.151107788,0.0,154.720443726,129.666244507,\"631T\",16,7,7,7,04,00,20,23*e5359168\n\t", "DUALANTENNAHEADINGA,USB3,0,49.5,FINESTEERING,2107,283328.400,02000000,d426,15824;SOL_COMPUTED,L1_FLOAT,-1.000000000,233.630966187,67.887474060,0.0,142.421936035,104.273208618,\"631T\",16,7,7,7,04,00,20,23*adc689dc\n\t", "INSPVAXA,USB3,0,47.5,FINESTEERING,2107,283329.450,02000000,471d,15824;INS_ALIGNMENT_COMPLETE,INS_RTKFIXED,37.37117634978,126.72305311232,7.7998,22.3000,0.0862,-0.3020,-0.0280,-0.761140788,-1.083777551,279.913760721,0.4381,0.2959,0.5691,0.1130,0.0927,0.0780,0.0968,0.1018,4.9666,0f000001,0*14477745\n\t", "DUALANTENNAHEADINGA,USB3,0,47.5,FINESTEERING,2107,283329.900,02000000,d426,15824;SOL_COMPUTED,L1_FLOAT,-1.000000000,242.466461182,68.906974792,0.0,305.866271973,174.467803955,\"631T\",16,7,7,7,04,00,20,23*70416e5a\n\t", "DUALANTENNAHEADINGA,USB3,0,45.5,FINESTEERING,2107,283330.400,02000000,d426,15824;SOL_COMPUTED,L1_FLOAT,-1.000000000,253.717498779,60.920593262,0.0,360.000000000,168.553268433,\"631T\",16,8,8,7,04,00,20,23*61124d9e\n\t", "DUALANTENNAHEADINGA,USB3,0,49.5,FINESTEERING,2107,283331.400,02000000,d426,15824;SOL_COMPUTED,L1_FLOAT,-1.000000000,237.639099121,66.545394897,0.0,164.585220337,123.074584961,\"631T\",15,7,7,7,04,00,20,23*2287d710\n\t", "DUALANTENNAHEADINGA,USB3,0,47.5,FINESTEERING,2107,283332.400,02000000,d426,15824;SOL_COMPUTED,L1_FLOAT,-1.000000000,240.635864258,62.019580841,0.0,147.512512207,88.501113892,\"631T\",15,8,8,7,04,00,20,23*1b578ca8\n\t", "DUALANTENNAHEADINGA,USB3,0,47.5,FINESTEERING,2107,283332.900,02000000,d426,15824;SOL_COMPUTED,L1_FLOAT,-1.000000000,240.870727539,61.885963440,0.0,149.317565918,88.725570679,\"631T\",15,8,8,7,04,00,20,23*f5ccc36e\n\t", "DUALANTENNAHEADINGA,USB3,0,47.0,FINESTEERING,2107,283333.900,02000000,d426,15824;SOL_COMPUTED,L1_FLOAT,-1.000000000,249.436477661,59.643127441,0.0,267.978637695,142.511169434,\"631T\",15,8,8,6,04,00,20,23*60a51aa1\n\t", "INSPVAXA,USB3,0,48.0,FINESTEERING,2107,283336.450,02008000,471d,15824;INS_ALIGNMENT_COMPLETE,INS_RTKFIXED,37.37118062962,126.72303171077,7.8093,22.3000,0.0910,-0.2726,-0.0070,-0.431620685,-0.601507753,279.754896357,0.4400,0.2962,0.5694,0.1129,0.0927,0.0780,0.0968,0.1018,4.9757,0f000001,0*323f8ead\n\t", "INSPVAXA,USB3,0,48.0,FINESTEERING,2107,283336.950,02008000,471d,15824;INS_ALIGNMENT_COMPLETE,INS_RTKFIXED,37.37118094970,126.72303018769,7.8089,22.3000,0.0850,-0.2634,-0.0148,-0.368097924,-0.496074380,279.888293307,0.4400,0.2962,0.5694,0.1129,0.0927,0.0780,0.0968,0.1018,4.9757,0f000001,0*6cd4e320\n\t", "INSPVAXA,USB3,0,49.0,FINESTEERING,2107,283337.450,02008000,471d,15824;INS_ALIGNMENT_COMPLETE,INS_RTKFIXED,37.37118121756,126.72302900978,7.8099,22.3000,0.0919,-0.3084,-0.0188,-0.391974632,-0.310525962,279.833764071,0.4417,0.2966,0.5697,0.1134,0.0928,0.0781,0.0968,0.1018,4.9771,0f000001,0*732111a1\n\t", "DUALANTENNAHEADINGA,USB3,0,49.0,FINESTEERING,2107,283337.900,02008000,d426,15824;SOL_COMPUTED,L1_FLOAT,-1.000000000,237.924728394,61.700553894,0.0,151.721710205,100.643135071,\"631T\",14,6,6,5,04,00,20,03*b8043138\n\t", "DUALANTENNAHEADINGA,USB3,0,50.0,FINESTEERING,2107,283338.400,02008000,d426,15824;SOL_COMPUTED,L1_FLOAT,-1.000000000,237.905731201,60.774238586,0.0,143.960494995,94.373596191,\"631T\",14,6,6,5,04,00,20,03*a8a19996\n\t", "INSPVAXA,USB3,0,50.0,FINESTEERING,2107,283338.950,02008000,471d,15824;INS_ALIGNMENT_COMPLETE,INS_RTKFIXED,37.37118224254,126.72302419522,7.8081,22.3000,0.0973,-0.2877,-0.0182,-0.386859897,-0.840656461,280.267328107,0.4433,0.2968,0.5700,0.1133,0.0930,0.0781,0.0968,0.1018,4.9781,0f000001,0*f46e19c3\n\t", "INSPVAXA,USB3,0,47.5,FINESTEERING,2107,283339.950,02000000,471d,15824;INS_ALIGNMENT_COMPLETE,INS_RTKFIXED,37.37118290995,126.72302108241,7.8055,22.3000,0.1047,-0.2801,-0.0151,-0.377109239,-0.859566836,280.447677121,0.4440,0.2973,0.5704,0.1133,0.0931,0.0781,0.0968,0.1018,4.9788,0f000001,0*ab964f25\n\t", "INSPVAXA,USB3,0,49.5,FINESTEERING,2107,283340.450,02000000,471d,15824;INS_ALIGNMENT_COMPLETE,INS_RTKFIXED,37.37118325232,126.72301952699,7.8038,22.3000,0.1007,-0.2812,-0.0170,-0.234742930,-0.655419935,280.541349843,0.4439,0.2974,0.5704,0.1133,0.0930,0.0781,0.0969,0.1018,4.9791,0f000001,0*59bc90eb\n\t", "DUALANTENNAHEADINGA,USB3,0,49.5,FINESTEERING,2107,283340.900,02000000,d426,15824;SOL_COMPUTED,NARROW_FLOAT,-1.000000000,267.637573242,68.984275818,0.0,360.000000000,180.000000000,\"631T\",17,6,6,5,04,00,20,03*859e1115\n\t", "INSPVAXA,USB3,0,44.0,FINESTEERING,2107,283341.950,02000000,471d,15824;INS_ALIGNMENT_COMPLETE,INS_RTKFIXED,37.37118432229,126.72301480701,7.8000,22.3000,0.1087,-0.2890,-0.0241,-0.323004853,-0.539804569,280.777320682,0.4437,0.2973,0.5706,0.1133,0.0929,0.0781,0.0969,0.1018,4.9792,0f000001,0*d82bda2e\n\t", "INSPVAXA,USB3,0,46.5,FINESTEERING,2107,283342.450,02000000,471d,15824;INS_ALIGNMENT_COMPLETE,INS_RTKFIXED,37.37118468084,126.72301322867,7.7994,22.3000,0.1106,-0.2869,-0.0271,-0.331140922,-0.546506458,280.773428519,0.4432,0.2972,0.5705,0.1132,0.0928,0.0781,0.0969,0.1018,4.9794,0f000001,0*c730c292\n\t", "INSPVAXA,USB3,0,46.5,FINESTEERING,2107,283342.950,02000000,471d,15824;INS_ALIGNMENT_COMPLETE,INS_RTKFIXED,37.37118504719,126.72301165338,7.7988,22.3000,0.1101,-0.2944,-0.0310,-0.265542746,-0.516192724,280.711326295,0.4432,0.2972,0.5705,0.1132,0.0928,0.0781,0.0969,0.1018,4.9794,0f000001,0*2bc99236\n\t", "INSPVAXA,USB3,0,46.0,FINESTEERING,2107,283343.450,02000000,471d,15824;INS_ALIGNMENT_COMPLETE,INS_RTKFIXED,37.37118540426,126.72301007829,7.7983,22.3000,0.1044,-0.2953,-0.0281,-0.322294329,-0.503749733,280.647452797,0.4438,0.2974,0.5709,0.1134,0.0929,0.0781,0.0970,0.1019,4.9802,0f000001,0*02b1cd5a\n\t", "INSPVAXA,USB3,0,46.0,FINESTEERING,2107,283343.950,02000000,471d,15824;INS_ALIGNMENT_COMPLETE,INS_RTKFIXED,37.37118578208,126.72300848824,7.7969,22.3000,0.1004,-0.2946,-0.0156,-0.222818059,-0.457044494,280.483100024,0.4438,0.2974,0.5709,0.1134,0.0929,0.0781,0.0970,0.1019,4.9802,0f000001,0*af3033cd\n\t", "INSPVAXA,USB3,0,45.0,FINESTEERING,2107,283344.450,02000000,471d,15824;INS_ALIGNMENT_COMPLETE,INS_RTKFIXED,37.37118614793,126.72300689991,7.7943,22.3000,0.0993,-0.2872,-0.0172,-0.186993521,-0.511161636,280.230119633,0.4441,0.2974,0.5711,0.1134,0.0928,0.0781,0.0970,0.1019,4.9812,0f000001,0*b466b7e8\n\t", "INSPVAXA,USB3,0,45.0,FINESTEERING,2107,283344.950,02000000,471d,15824;INS_ALIGNMENT_COMPLETE,INS_RTKFIXED,37.37118650785,126.72300530954,7.7912,22.3000,0.0978,-0.2991,-0.0150,-0.269374143,-0.498749475,279.993433962,0.4441,0.2974,0.5711,0.1134,0.0928,0.0781,0.0970,0.1019,4.9812,0f000001,0*f4f3a5d7\n\t", "INSPVAXA,USB3,0,49.0,FINESTEERING,2107,283345.450,02000000,471d,15824;INS_ALIGNMENT_COMPLETE,INS_RTKFIXED,37.37118684878,126.72300372907,7.7899,22.3000,0.0930,-0.2956,-0.0147,-0.404221578,-0.693160058,279.694670090,0.4438,0.2972,0.5711,0.1134,0.0928,0.0781,0.0970,0.1019,4.9825,0f000001,0*306daf1e\n\t", "INSPVAXA,USB3,0,49.0,FINESTEERING,2107,283345.950,02000000,471d,15824;INS_ALIGNMENT_COMPLETE,INS_RTKFIXED,37.37118719722,126.72300213566,7.7889,22.3000,0.0945,-0.2844,-0.0103,-0.444285686,-0.741424301,279.319475907,0.4438,0.2972,0.5711,0.1134,0.0928,0.0781,0.0970,0.1019,4.9825,0f000001,0*d5c67081\n\t", "INSPVAXA,USB3,0,45.5,FINESTEERING,2107,283346.450,02000000,471d,15824;INS_ALIGNMENT_COMPLETE,INS_RTKFIXED,37.37118745204,126.72300097325,7.7876,22.3000,0.0956,-0.2876,-0.0148,-0.514894680,-0.480743758,278.986298177,0.4452,0.2974,0.5713,0.1136,
